vi "ResetSettingControl.vi"(10 "This VI":refnum<vi>, 11 "MainMenu_In":refnum<vi>) -> ()   [LabVIEW 2013]
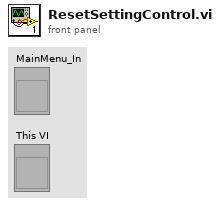
[diagram p1: front panel]
types:
  T1 = cluster{"Measurement":bool, "Save Data":bool, "LoadSetting":bool, "Save setting":bool, "Reset setting":bool, "Exit":bool}
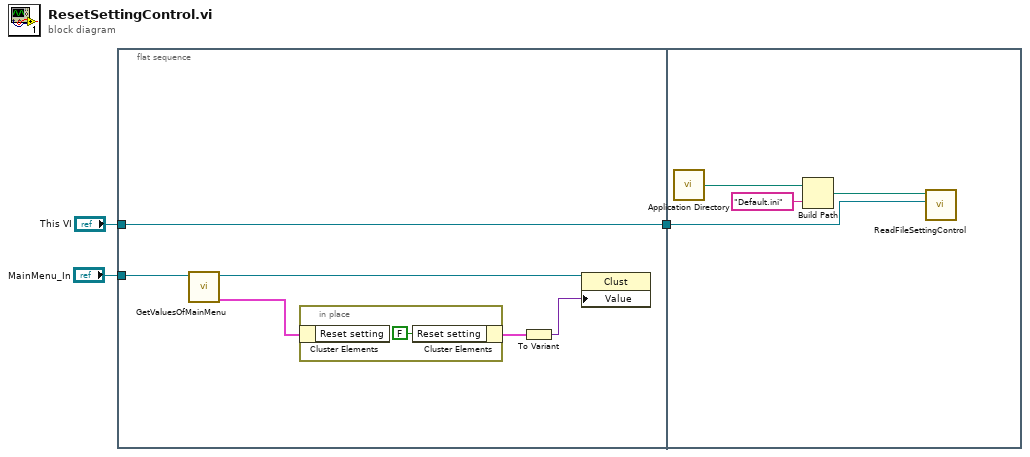
[diagram p0: block diagram]
diagram:
  n1 = flat-sequence {
    tunnel: "This VI" -> [w9]
    tunnel: [w9] -> w3
    tunnel: "MainMenu_In" -> [w8]
    tunnel: w3 -> [w11]
    frame #0 {
      n2 = call "GetValuesOfMainMenu.vi"("MainMenu_In"=w8) -> ("ValuesOfMainMenu"=w7:T1, "MainMenu_Out"=w6:refnum<vi>)  [unwired: 9 in]
      n3 = in-place {
        n4 = in-place-cluster #1(w7) -> ()  [unwired: 1 out]
        n5 = in-place-cluster #1("Reset setting"=FALSE ("LoadSetting")) -> (w5:T1)
      }
      n6 = To Variant(anything=w5) -> (Variant=w4:variant)
      n7 = property class="Clust"(reference=w6, "Value"=w4) -> ()  [unwired: 1 in, 2 out]
    }
    frame #1 {
      n8 = call <vilib>:"Application Directory.vi"() -> ("Application Directory"=w13:path)
      n9 = Build Path(base path=w13, name or relative path="Default.ini") -> (appended path=w12:path)
      n10 = call "ReadFileSettingControl.vi"("ThisVI_In"=w11, "Path to was selected by user"=w12) -> ()  [unwired: 9 in, 1 out]
    }
  }
